vi "start.vi"(8 "error in (no error)":errorcluster, 11 "FPGAWrapperDL090211Galvo in":refnum<class "FPGAWrapperDL090211Galvo_grabber.lvclass">) -> (0 "error out":errorcluster, 3 "FPGAWrapperDL090211Galvo out":refnum<class "FPGAWrapperDL090211Galvo_grabber.lvclass">)   [LabVIEW 2010, in "FPGAWrapperDL090211Galvo_grabber.lvclass"]
uses:
  FPGAWrapperDL090211Galvo_grabber.lvclass
  type definitions/command_enum.ctl
  class_data.vi
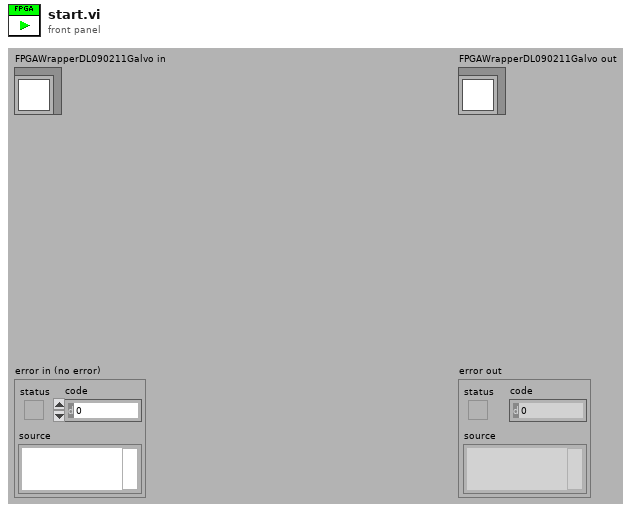
[diagram p1: front panel]
types:
  T1 = typedef "command_enum.ctl" = enum16{"NULL", "update", "start", "stop", "reset", "shut-down"}
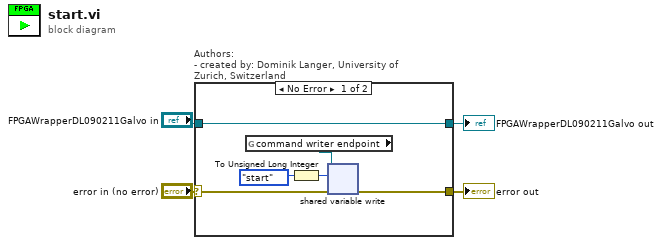
[diagram p0: block diagram]
diagram:
  n1 = case "Authors: \n- created by: Dominik Langer, University of Zurich, Switzerland" shown="No Error" "error in (no error)" {
    selector: "error in (no error)" -> [w9 w11]
    tunnel: "FPGAWrapperDL090211Galvo in" -> [w10 w12]
    tunnel: [w10 w12] -> w3
    tunnel: [w8 w11] -> w2
    frame No Error {
      n2 = global read "class_data.vi" "command writer endpoint"() -> (w5:refnum<k21>)
      n3 = To Unsigned Long Integer(number=command_enum."start" ("command")) -> (unsigned 32bit integer=w7:u32)
      n4 = shared-variable-write(w5, w9, w7) -> (w8:errorcluster)  [unwired: 1 in, 2 out]
    }
    frame Error {
    }
  }
  "error out" <- w2
  "FPGAWrapperDL090211Galvo out" <- w3
